vi "QPSK_Main.vi"() -> ()   [LabVIEW 2015]
uses:
  LabviewSubVI/RFConfig/StudentMsg.ctl
  LabviewSubVI/RFConfig/RF_Config.ctl
panel:
  out "纠正前星座图":cdb[](graph)
  out "当前帧接收信号波形(Q路)":dbl[](graph)
  out "当前帧发送信号波形(Q路)":dbl[](graph)
  out "相关峰波形图":dbl[](graph)
  out "总误码数":dbl
  out "总误码率":dbl
  out "当前帧误码数":dbl
  out "当前帧误码率":dbl
  in  "信噪比(dB)":u8=30 max=50 step=1
  out "当前帧接收信号波形(I路)":dbl[](graph)
  out "当前帧发送信号波形(I路)":dbl[](graph)
  in  "XSRP IP":string="192.168.1.167"
  in  "PC IP":string="192.168.1.181"
  in  "运行方式":enum16{"仿真系统", "真实系统"}(ring)
  out "纠正后星座图":cdb[](graph)
  out "发送星座图":cdb[](graph)
  out "接收语音信号波形":dbl[](graph)
  out "发送语音信号波形":dbl[](graph)
  out "当前帧号":dbl
  out "当前帧CRC Flag":dbl
  in  "接收语音文件写入路径":path=path "C:/Users/mm/Desktop/work/Comprehensive Design/Lab02 QPSK communication system/01 TeacherVersion/Matlabcode/recvsound.wav"
  in  "发送语音文件读取路径":path=path "C:/Users/mm/Desktop/work/Comprehensive Design/Lab02 QPSK communication system/01 TeacherVersion/Matlabcode/Windows XP.wav"
  in  "?":T1={"发射频率"=900000000, "发射衰减"=44, "接收频率"=900000000, "接收增益"=12, "接收通道"=enum."RxCh1", "发射通道"=enum."TxCh1"} {"接收增益" max=40 format="%.0fdB"; "接收频率" min=70000000 max=6000000000 format="%.6pHz"; "发射衰减" max=90 format="%.0fdB"; "发射频率" min=70000000 max=6000000000 format="%.6pHz"}
  out "实验学生信息":T2={"姓名"="XXX\n", "学号"="XXX", "班级"="XXX", "学校"="XXX"}
  # "基于XSRP软件无线电平台的QPSK无线传输系统"
  # "实验参数设置"
  # "注：总误码率和总误码数运行完成后计算显示"
  # "实验学生信息"
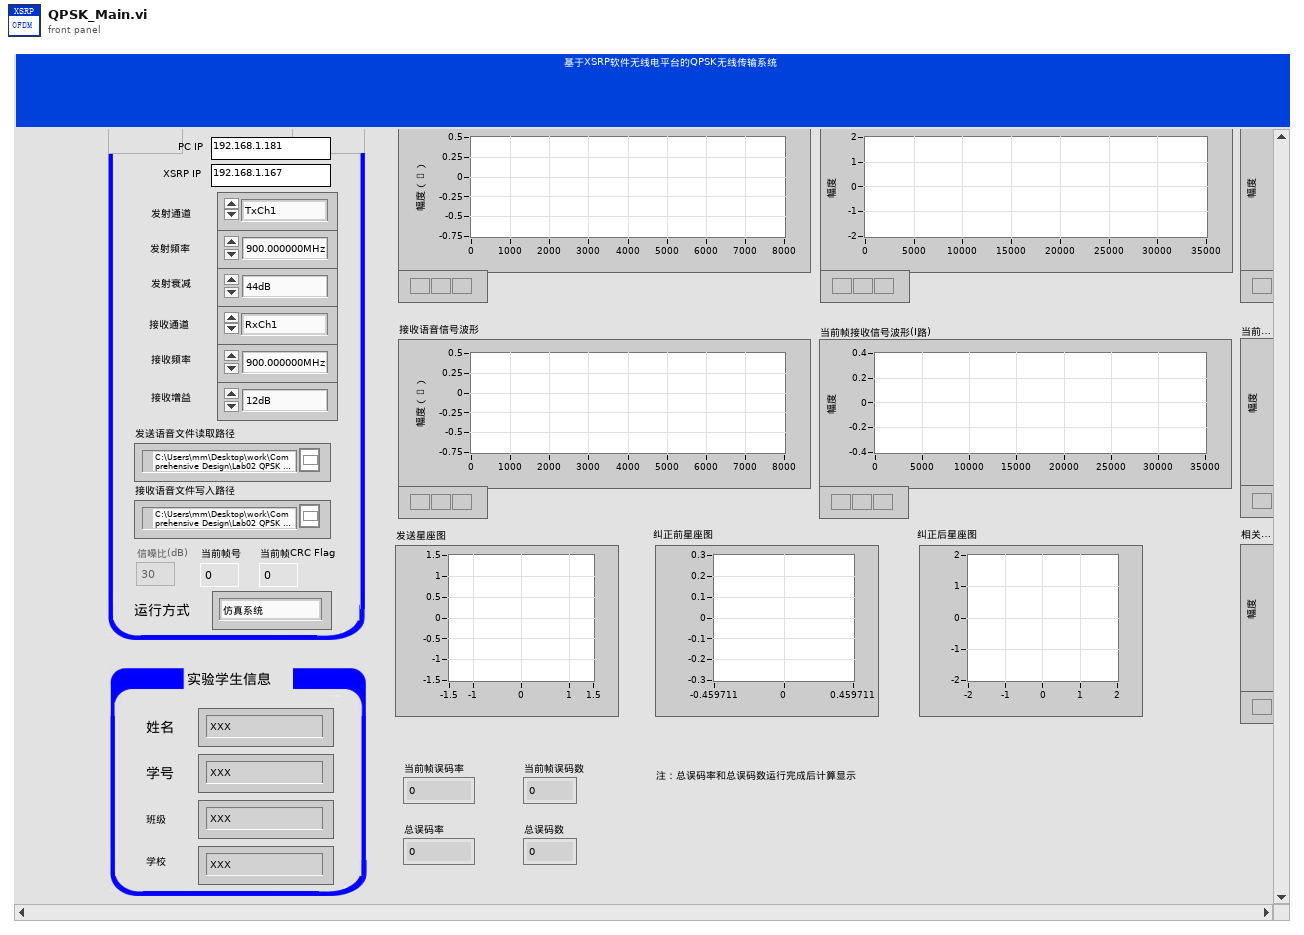
[diagram p1: front panel]
types:
  T1 = typedef "RF_Config.ctl" = cluster{"发射频率":u64, "发射衰减":u8, "接收频率":u64, "接收增益":u8, "接收通道":enum16{"RxCh1", "RxCh2"}, "发射通道":enum16{"TxCh1", "TxCh2"}}
  T2 = typedef "StudentMsg.ctl" = cluster{"姓名":string, "学号":string, "班级":string, "学校":string}
  T3 = enum8{"Enabled", "Disabled", "Disabled and Grayed Out"}
  T4 = cluster{"接收通道":enum16{"RxCh1", "RxCh2"}, "接收频率":u32, "接收增益":u8}
  T5 = cluster{"发射通道":enum16{"TxCh1", "TxCh2"}, "发射频率":u32, "发射衰减":u8}
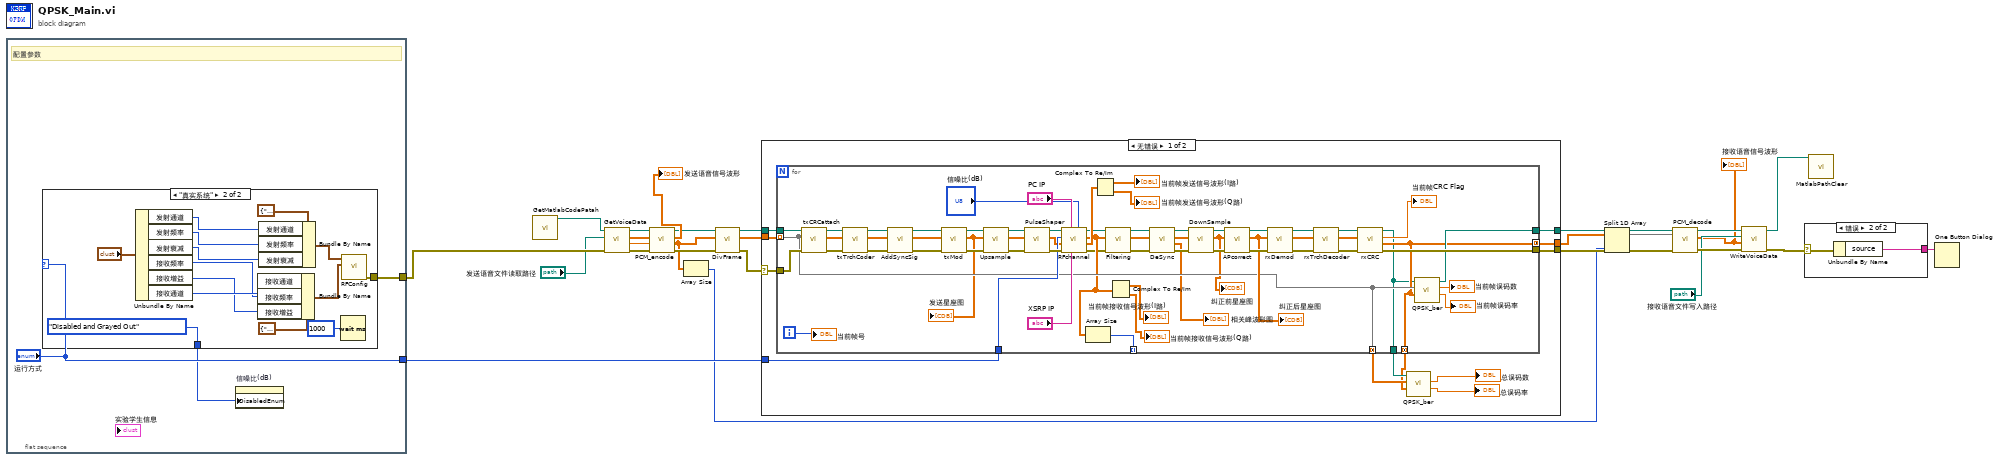
[diagram p0: block diagram]
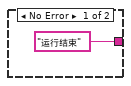
[diagram p3: hidden frame]
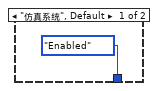
[diagram p4: hidden frame]
diagram:
  n1 = flat-sequence {
    tunnel: [w30] -> w27
    tunnel: ["运行方式"] -> w11
    frame #0 {
      # "配置参数"
      n2 = case shown="\"真实系统\"" "运行方式" {
        tunnel: [_ w34] -> w30
        tunnel: [T3."Enabled" ("Disabled") T3."Disabled and Grayed Out" ("Disabled")] -> w28
        frame "仿真系统", Default {
        }
        frame "真实系统" {
          n3 = Unbundle By Name("?") -> ("发射通道"=w42:enum16{"TxCh1", "TxCh2"}, "发射频率"=w41:u64, "发射衰减"=w40:u8, "接收频率"=w36:u64, "接收增益"=w37:u8, "接收通道"=w38:enum16{"RxCh1", "RxCh2"})
          n4 = Bundle By Name(cluster=T4 {"接收通道"=enum."RxCh1", "接收频率"=0, "接收增益"=0} ("接收参数设置"), "接收通道"=w38, "接收频率"=w36, "接收增益"=w37) -> (w35:T4)
          n5 = Bundle By Name(cluster=T5 {"发射通道"=enum."TxCh1", "发射频率"=0, "发射衰减"=0} ("发射参数设置"), "发射通道"=w42, "发射频率"=w41, "发射衰减"=w40) -> (w44:T5)
          n6 = Wait (ms)(milliseconds to wait=u32 1000) -> ()  [unwired: 1 out]
          n7 = call "RFConfig.vi"("接收参数设置"=w35, "发射参数设置"=w44) -> ("error out"=w34:errorcluster)  [unwired: 9 in]
        }
      }
      n8 = property on="信噪比(dB)" class="DigNum (严格)"("DisabledEnum"=w28) -> ()  [unwired: 2 in, 2 out]
    }
  }
  n9 = call "GetMatlabCodePatah.vi"() -> ("MatlabCodePath"=w16:path)  [unwired: 11 in]
  n10 = call "GetVoiceData.vi"("error in"=w27, "filePath"="发送语音文件读取路径", "Path In"=w16) -> ("error out"=w26:errorcluster, "Fs"=w20:dbl, "voiceData"=w13:dbl[], "Path Out"=w21:path)  [unwired: 5 in]
  n11 = call "PCM_encode.vi"("error in"=w26, "Fs"=w20, "voiceData"=w13, "Path In"=w21) -> ("error out"=w6:errorcluster, "encode_data"=w4:dbl[], "sampleData"=→"发送语音信号波形":dbl[], "Path Out"=w9:path)  [unwired: 4 in]
  n12 = Array Size(array=w4) -> (size(s)=w3:i32)
  n13 = call "DivFrame.vi"("error in"=w6, "encode_data"=w4, "Path In"=w9) -> ("error out"=w5:errorcluster, "FreData"=w7:dbl[][], "Path Out"=w8:path)  [unwired: 5 in, 1 out]
  n14 = case shown="无错误" w5 {
    selector: w5 -> [w52 w119]
    tunnel: [w57 w119] -> w25
    tunnel: w7 -> [w56 _]
    tunnel: w8 -> [w55 w120]
    tunnel: [w54 _] -> w2
    tunnel: [w53 w120] -> w19
    tunnel: w11 -> [w51 _]
    frame No Error {
      n15 = for {
        tunnel: [w81] -> w54 mode=concatenating
        tunnel: w56 -> [w82] mode=indexing
        tunnel: [w116] -> w57
        tunnel: w52 -> [w106]
        tunnel: w55 -> [w105]
        tunnel: [w88] -> w53
        tunnel: w51 -> [w94]
        tunnel: [w85] -> _ mode=indexing
        tunnel: [w82] -> w50 mode=concatenating
        tunnel: [w81] -> w48 mode=concatenating
        tunnel: [w80] -> w49
        i -> [w96]
        n16 = call "txCRCattach.vi"("error in"=w106, "inputData"=w82, "Path In"=w105) -> ("error out"=w118:errorcluster, "out_data"=w103:dbl[], "Path Out"=w104:path)  [unwired: 6 in]
        n17 = call "txTrchCoder.vi"("error in"=w118, "input_data"=w103, "Path In"=w104) -> ("error out"=w63:errorcluster, "out_data"=w65:dbl[], "Path Out"=w67:path)  [unwired: 6 in]
        n18 = call "AddSyncSig.vi"("error in"=w63, "inputData"=w65, "Path In"=w67) -> ("error out"=w62:errorcluster, "out_data"=w64:cdb[], "Path Out"=w66:path)  [unwired: 6 in]
        n19 = call "txMod.vi"("error in"=w62, "inputData"=w64, "Path In"=w66) -> ("error out"=w70:errorcluster, "out_data"=w69:cdb[], "Path Out"=w68:path)  [unwired: 6 in]
        "发送星座图" <- w69
        n20 = call "Upsample.vi"("error in"=w70, "inputData"=w69, "Path In"=w68) -> ("error out"=w71:errorcluster, "out_data"=w72:cdb[], "Path Out"=w73:path)  [unwired: 6 in]
        n21 = call "PulseShaper.vi"("error in"=w71, "inputData"=w72, "Path In"=w73) -> ("error out"=w111:errorcluster, "out_data"=w84:cdb[], "Path Out"=w107:path)  [unwired: 6 in]
        n22 = call "RFchannel.vi"("snr"="信噪比(dB)", "xsrpip"="XSRP IP", "pcip"="PC IP", "error in (no error)"=w111, "out_data"=w84, "运行方式"=w94, "Path In"=w107) -> ("error out"=w75:errorcluster, "txdataIQ"=w83:cdb[], "rxdataIQ"=w77:cdb[], "Path Out"=w79:path)  [unwired: 1 in]
        n23 = Array Size(array=w77) -> (size(s)=w85:i32)
        n24 = Complex To Re/Im(x + iy=w83) -> (x=→"当前帧发送信号波形(I路)":dbl[], y=→"当前帧发送信号波形(Q路)":dbl[])
        n25 = call "Filtering.vi"("error in (no error)"=w75, "input_data"=w77, "PathIn"=w79) -> ("error out"=w74:errorcluster, "out_data"=w76:cdb[], "PathOut"=w78:path)  [unwired: 6 in]
        n26 = Complex To Re/Im(x + iy=w77) -> (x=→"当前帧接收信号波形(I路)":dbl[], y=→"当前帧接收信号波形(Q路)":dbl[])
        n27 = call "DeSync.vi"("error in"=w74, "inputData"=w76, "Path In"=w78) -> ("error out"=w110:errorcluster, "modScCorr"=→"相关峰波形图":dbl[], "out_data"=w101:cdb[], "Path Out"=w102:path)  [unwired: 5 in]
        n28 = call "DownSample.vi"("error in"=w110, "inputData"=w101, "Path In"=w102) -> ("error out"=w109:errorcluster, "out_data"=w58:cdb[], "Path Out"=w113:path)  [unwired: 6 in]
        "纠正前星座图" <- w58
        n29 = call "APcorrect.vi"("error in"=w109, "inputData"=w58, "Path In"=w113) -> ("error out"=w108:errorcluster, "out_data"=w95:cdb[], "Path Out"=w112:path)  [unwired: 6 in]
        "纠正后星座图" <- w95
        n30 = call "rxDemod.vi"("error in"=w108, "inputData"=w95, "Path In"=w112) -> ("error out"=w114:errorcluster, "outData"=w99:dbl[], "Path Out"=w100:path)  [unwired: 6 in]
        n31 = call "rxTrchDecoder.vi"("error in"=w114, "inputData"=w99, "Path In"=w100) -> ("error out"=w117:errorcluster, "out_data"=w98:dbl[], "Path Out"=w115:path)  [unwired: 6 in]
        n32 = call "rxCRC.vi"("error in"=w117, "inputData"=w98, "Path In"=w115) -> ("error out"=w116:errorcluster, "out_data"=w81:dbl[], "CRC_flag"=→"当前帧CRC Flag":dbl, "Path Out"=w80:path)  [unwired: 5 in]
        n33 = call "QPSK_ber.vi"("rxbit"=w81, "txbit"=w82, "Path In"=w80) -> ("ber"=→"当前帧误码率":dbl, "errnum"=→"当前帧误码数":dbl, "Path Out"=w88:path)  [unwired: 5 in, 1 out]
        "当前帧号" <- w96
      }
      n34 = call "QPSK_ber.vi"("rxbit"=w48, "txbit"=w50, "Path In"=w49) -> ("ber"=→"总误码率":dbl, "errnum"=→"总误码数":dbl)  [unwired: 5 in, 2 out]
    }
    frame Error {
    }
  }
  n35 = Split 1D Array(array=w2, index=w3) -> (first subarray=w1:dbl[])  [unwired: 1 out]
  n36 = call "PCM_decode.vi"("error in"=w25, "inputData"=w1, "Path In"=w19) -> ("error out"=w24:errorcluster, "outData"=w12:dbl[], "Path Out"=w18:path)  [unwired: 6 in]
  "接收语音信号波形" <- w12
  n37 = call "WriteVoiceData.vi"("error in"=w24, "input_data"=w12, "filePath"="接收语音文件写入路径", "Path In"=w18) -> ("error out"=w23:errorcluster, "Path Out"=w17:path)  [unwired: 5 in, 1 out]
  n38 = case shown="错误" w23 {
    selector: w23 -> [_ w123]
    tunnel: ["运行结束" ("source") w122] -> w22
    frame No Error {
    }
    frame Error {
      n39 = Unbundle By Name(w123) -> ("source"=w122:string)
    }
  }
  n40 = call "MatlabPathClear.vi"("Path"=w17) -> ()  [unwired: 10 in, 1 out]
  n41 = One Button Dialog(message=w22) -> ()  [unwired: 1 in, 1 out]
